vi "Filter1DArray.vi"(10 "Keep?":bool[](array[boolean]), 11 "Array":bool[](array[boolean])) -> (3 "Filtered Array":bool[](array[boolean]))   [LabVIEW 2021, in "Bananas.lvlib" / "Pips.lvclass"]
uses:
  Pips.lvclass
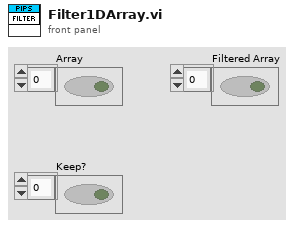
[diagram p1: front panel]
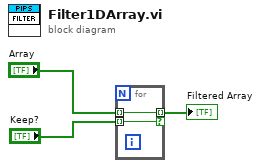
[diagram p0: block diagram]
diagram:
  n1 = for {
    tunnel: [w5] -> w2 mode=indexing if=w4
    tunnel: "Array" -> [w5] mode=indexing
    tunnel: "Keep?" -> [w4] mode=indexing
  }
  "Filtered Array" <- w2
